vi "COMTRADE Read Private Inf (All Entries).vi"(8 "error in (no error)":errorcluster, 9 "section name":string, 10 "manufacturer name":string, 11 "task in":T1={"file refnums"=[], "Data Object"=refnum, "config info"={"station_name"="", "rec_dev_id"="", "rev_year"=1999.0, "TT"=0, "##A"=0, "##D"=0, "analog channel info"=[], "status channel info"=[], "lf"=50.0, "nrates"=0, "samp info"=[], "initial timestamp"=timestamp(0 s since 1904-01-01), "trigger timestamp"=timestamp(0 s since 1904-01-01), "ft"=enum."Binary", "timemult"=1.0}, "public inf content"={"Source"="", "Record Type"=enum."Unknown", "Phase ID"="", "Event Description"="", "Device ID"="", "Distance of Fault"=-1.0, "Distance Unit"=enum."Miles", "Max_Current"=inf, "Min_Current"=-inf, "Max_Voltage"=inf, "Min_Voltage"=-inf, "EventNoteCount"=0, "Event Information"=[]}, "private inf content"=[], "internal buffers"={"start index"=1, "config to public inf"=enum."disabled", "static config info"="", "static file_des record inf"="", "static file_des channel inf"="", "public inf"="", "private inf"=""}} {"public inf content"."Event Information"."min sample number" max=9999999999; "public inf content"."Event Information"."max sample number" max=9999999999; "config info"."nrates" max=999; "config info"."status channel info"."Dn" min=1 max=999999; "config info"."analog channel info"."An" min=1 max=999999; "config info"."trigger timestamp" format="%<%H:%M:%S%6u\n%d/%m/%Y>T"; "config info"."initial timestamp" format="%<%H:%M:%S%6u\n%d/%m/%Y>T"; "config info"."##D" max=999999; "config info"."##A" max=999999; "config info"."TT" min=1 max=999999; "config info"."rev_year" min=1999.0 max=1999.0}) -> (0 "error out":errorcluster, 1 "entry values":string[](array[string]), 2 "entry names":string[](array[string]), 3 "task out":T1={"file refnums"=[], "Data Object"=refnum, "config info"={"station_name"="", "rec_dev_id"="", "rev_year"=1999.0, "TT"=0, "##A"=0, "##D"=0, "analog channel info"=[], "status channel info"=[], "lf"=50.0, "nrates"=0, "samp info"=[], "initial timestamp"=timestamp(0 s since 1904-01-01), "trigger timestamp"=timestamp(0 s since 1904-01-01), "ft"=enum."Binary", "timemult"=1.0}, "public inf content"={"Source"="", "Record Type"=enum."Unknown", "Phase ID"="", "Event Description"="", "Device ID"="", "Distance of Fault"=-1.0, "Distance Unit"=enum."Miles", "Max_Current"=inf, "Min_Current"=-inf, "Max_Voltage"=inf, "Min_Voltage"=-inf, "EventNoteCount"=0, "Event Information"=[]}, "private inf content"=[], "internal buffers"={"start index"=1, "config to public inf"=enum."disabled", "static config info"="", "static file_des record inf"="", "static file_des channel inf"="", "public inf"="", "private inf"=""}} {"public inf content"."Event Information"."min sample number" max=9999999999; "public inf content"."Event Information"."max sample number" max=9999999999; "config info"."nrates" max=999; "config info"."status channel info"."Dn" min=1 max=999999; "config info"."analog channel info"."An" min=1 max=999999; "config info"."trigger timestamp" format="%<%H:%M:%S%6u\n%d/%m/%Y>T"; "config info"."initial timestamp" format="%<%H:%M:%S%6u\n%d/%m/%Y>T"; "config info"."##D" max=999999; "config info"."##A" max=999999; "config info"."TT" min=1 max=999999; "config info"."rev_year" min=1999.0 max=1999.0})   [LabVIEW 2013, in "NI_EP_COMTRADE.lvlib"]
doc: "Reads information from the private sections of the optionally specified .inf file. You must set <B>open mode</B> to Open (read only) in the COMTRADE Open VI to open the .inf file. Otherwise this VI returns an error."
uses:
  <vilib>/addons/Electrical Power/File IO/NI_EP_COMTRADE.lvlib
  <vilib>/addons/Electrical Power/File IO/COMTRADE/typedefs/ep_Task.ctl
  <vilib>/addons/Electrical Power/File IO/COMTRADE/typedefs/ep_Config Info.ctl
  <vilib>/addons/Electrical Power/File IO/COMTRADE/typedefs/ep_Analog Channel Info.ctl
  <vilib>/addons/Electrical Power/File IO/COMTRADE/typedefs/ep_Status Channel Info.ctl
  <vilib>/addons/Electrical Power/File IO/COMTRADE/typedefs/ep_File Format.ctl
  <vilib>/addons/Electrical Power/File IO/COMTRADE/typedefs/ep_Public Inf Content.ctl
  <vilib>/addons/Electrical Power/File IO/COMTRADE/typedefs/ep_Public Event Inf.ctl
  <vilib>/addons/Electrical Power/File IO/COMTRADE/typedefs/ep_Private Inf Content.ctl
  <vilib>/Platform/storage/Storage.llb/Get Property (Storage Refnums).vi
  <vilib>/Platform/storage/Storage.llb/Get Property (I32).vi
  <vilib>/Platform/storage/Storage.llb/Get Property (String).vi
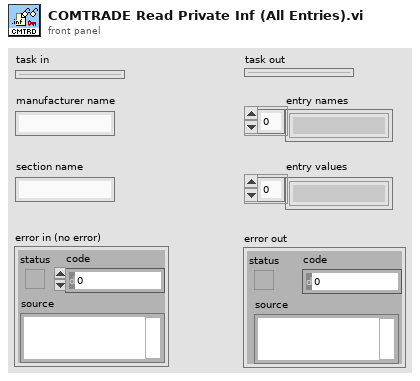
[diagram p1: front panel]
types:
  T1 = typedef "NI_EP_COMTRADE.lvlib/ep_Task.ctl" = cluster{"file refnums":refnum<file>[], "Data Object":refnum<k20>, "config info":T2, "public inf content":T6, "private inf content":T8, "internal buffers":cluster{"start index":u32, "config to public inf":enum16{"disabled", "enabled", "buffered"}, "static config info":string, "static file_des record inf":string, "static file_des channel inf":string, "public inf":string, "private inf":string}}
  T2 = typedef "NI_EP_COMTRADE.lvlib/ep_Config Info.ctl" = cluster{"station_name":string, "rec_dev_id":string, "rev_year":dbl, "TT":u32, "##A":u32, "##D":u32, "analog channel info":T3[], "status channel info":T4[], "lf":sgl, "nrates":u16, "samp info":cluster{"samp":sgl, "endsamp":u32}[], "initial timestamp":timestamp, "trigger timestamp":timestamp, "ft":T5, "timemult":sgl}
  T3 = typedef "NI_EP_COMTRADE.lvlib/ep_Analog Channel Info.ctl" = cluster{"An":u32, "ch_id":string, "ph":string, "ccbm":string, "uu":string, "a":sgl, "b":sgl, "skew":sgl, "min":i32, "max":i32, "primary":sgl, "secondary":sgl, "PS":enum16{"P", "S"}}
  T4 = typedef "NI_EP_COMTRADE.lvlib/ep_Status Channel Info.ctl" = cluster{"Dn":u32, "ch_id":string, "ph":string, "ccbm":string, "Y":bool}
  T5 = typedef "NI_EP_COMTRADE.lvlib/ep_File Format.ctl" = enum16{"ASCII", "Binary"}
  T6 = typedef "NI_EP_COMTRADE.lvlib/ep_Public Inf Content.ctl" = cluster{"Source":string, "Record Type":enum16{"Fault", "Unknown", "Misoperation", "Close", "Trip", "Reclose", "Power swing", "Simulation"}, "Phase ID":string, "Event Description":string, "Device ID":string, "Distance of Fault":dbl, "Distance Unit":enum16{"Miles", "Kilometers", "Percent of line", "Percent of setting", "Ohms"}, "Max_Current":dbl, "Min_Current":dbl, "Max_Voltage":dbl, "Min_Voltage":dbl, "EventNoteCount":u32, "Event Information":T7[]}
  T7 = typedef "NI_EP_COMTRADE.lvlib/ep_Public Event Inf.ctl" = cluster{"channel number":u32, "max value":dbl, "min value":dbl, "max sample number":u64, "min sample number":u64, "max sample text":string[], "min sample text":string[]}
  T8 = typedef "NI_EP_COMTRADE.lvlib/ep_Private Inf Content.ctl" = cluster{"Section Header":string, "Entry Names":string[], "Entry Values":string[]}[]
  T9 = typedef "usiProperty.ctl" = cluster{"object type":T10, "property name":string, "data type":T11}
  T10 = typedef "usiObjectType.ctl" = enum16{"File", "Channel Group", "Channel", "Unknown"}
  T11 = typedef "usiDataType.ctl" = enum16{"eNoTypeUsi", "eInt8Usi", "eInt16Usi", "eInt32Usi", "eInt64Usi", "eUInt8Usi", "eUInt16Usi", "eUInt32Usi", "eUInt64Usi", "eFloat32Usi", "eFloat64Usi", "- 0", "- 1", "- 2", "- 3", "- 4", "- 5", "- 6", "- 7", "- 8", "- 9", "eString8Usi", "eString16Usi", "eStringUsi", "eEnumUsi", "- 10", "- 11", "- 12", "- 13", "- 14", "eTimeUsi", "- 15", "- 16", "- 17", "- 18", "- 19", "- 20", "- 21", "- 22", "- 23", "eInstanceUsi", "eStoreUsi"}
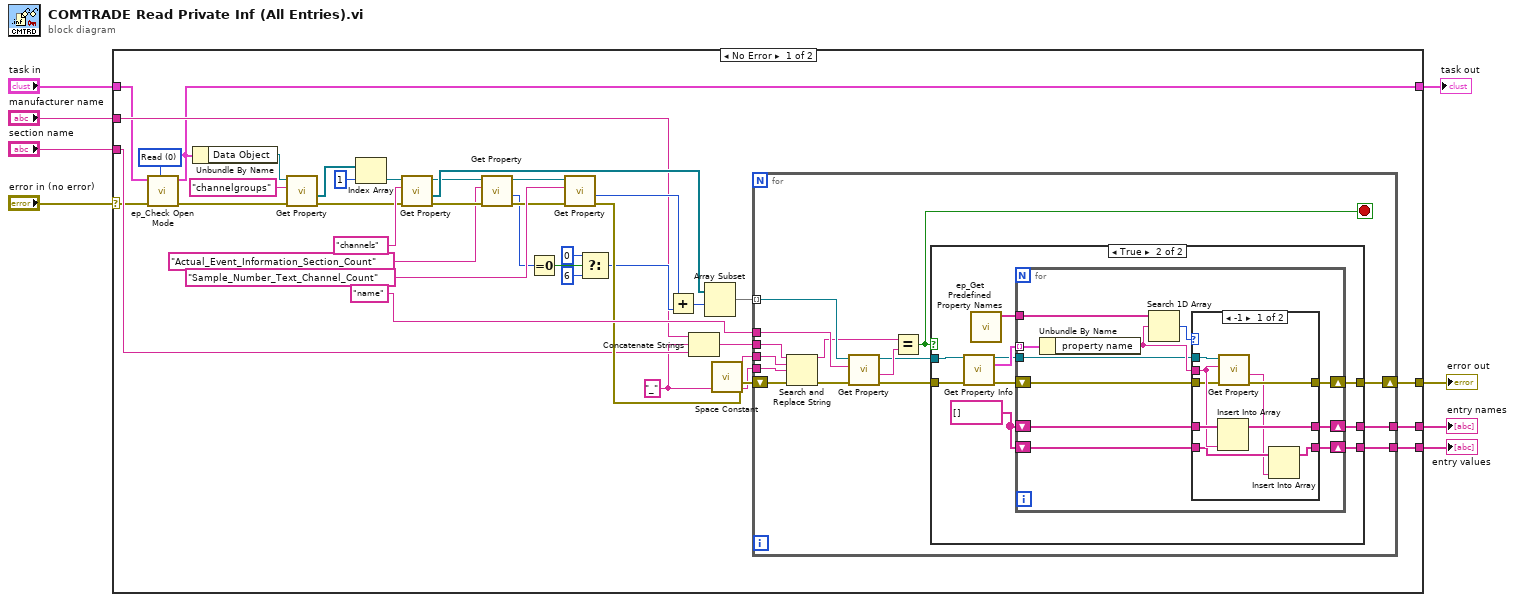
[diagram p0: block diagram]
diagram:
  n1 = case shown="No Error" "error in (no error)" {
    selector: "error in (no error)" -> [w12 w95]
    tunnel: "task in" -> [w10 w96]
    tunnel: [w9 w96] -> w3
    tunnel: [w29 w95] -> w7
    tunnel: "manufacturer name" -> [w18 _]
    tunnel: "section name" -> [w31 _]
    tunnel: [w15 _] -> w1
    tunnel: [w14 _] -> w2
    frame No Error {
      w13 = u16 0 items=["Read", "Write"] ("file type")
      w16 = "_" ("string")
      n2 = call <vilib>:"ep_Check Open Mode.vi"("expected mode"=w13, "error in (no error)"=w12, "task in"=w10) -> ("error out"=w11:errorcluster, "task out"=w9:T1)  [unwired: 7 in]
      n3 = Unbundle By Name(w9) -> ("Data Object"=w45:refnum<k20>)
      n4 = call-poly <vilib>:"Get Property.vi"("error in (no error)"=w11, "Property name"="channelgroups", "storage refnum"=w45) -> ("error out"=w35:errorcluster, "Value"=w44:refnum<k20>[])  [unwired: 6 in, 1 out]
      n5 = Index Array(array=w44, index=1) -> (element=w40:refnum<k20>)
      n6 = call-poly <vilib>:"Get Property.vi"("error in (no error)"=w35, "Property name"="channels", "storage refnum"=w40) -> ("error out"=w28:errorcluster, "Value"=w39:refnum<k20>[], "storage refnum out"=w20:refnum<k20>)  [unwired: 6 in]
      n7 = call-poly <vilib>:"Get Property.vi"("error in (no error)"=w28, "Property name"="Actual_Event_Information_Section_Count", "storage refnum"=w20) -> ("error out"=w27:errorcluster, "Value"=w24:i32, "storage refnum out"=w19:refnum<k20>)  [unwired: 6 in]
      n8 = Equal To 0?(x=w24) -> (x = 0?=w25:bool)
      n9 = call-poly <vilib>:"Get Property.vi"("error in (no error)"=w27, "Property name"="Sample_Number_Text_Channel_Count", "storage refnum"=w19) -> ("error out"=w32:errorcluster, "Value"=w37:i32)  [unwired: 6 in, 1 out]
      n10 = Select(t=0 ("index"), s=w25, f=6 ("index")) -> (s? t:f=w23:i32)
      n11 = Add(x=w37, y=w23) -> (x+y=w38:i32)
      n12 = Concatenate Strings(w18, w16, w31) -> (w30:string)
      n13 = Array Subset(array=w39, index=w38) -> (w34:refnum<k20>[])  [unwired: 1 in]
      n14 = call <vilib>:"Space Constant.vi"() -> ("String"=w17:string)
      n15 = for {
        tunnel: w34 -> [w60] mode=indexing
        tunnel: "name" ("Property name") -> [w59]
        shift-right: [w47] -> w29
        shift-left: w32 -> [w51]
        tunnel: w30 -> [w54]
        tunnel: w17 -> [w53]
        tunnel: w16 -> [w52]
        tunnel: [w48] -> w15
        tunnel: [w46] -> w14
        stop <- w55 stop-if-true
        n16 = Search and Replace String(input string=w54, search string=w53, replace string=w52, error in=w51) -> (result string=w49:string, error out=w50:errorcluster)  [unwired: 4 in, 2 out]
        n17 = call-poly <vilib>:"Get Property.vi"("error in (no error)"=w50, "Property name"=w59, "storage refnum"=w60) -> ("error out"=w56:errorcluster, "Value"=w58:string, "storage refnum out"=w57:refnum<k20>)  [unwired: 6 in]
        n18 = Equal?(x=w49, y=w58) -> (x = y?=w55:bool)
        n19 = case shown="True" w55 {
          tunnel: w57 -> [_ w68]
          tunnel: w56 -> [w61 w71]
          tunnel: [w61 w64] -> w47
          tunnel: [_ w63] -> w48
          tunnel: [_ w67] -> w46
          frame False {
          }
          frame True {
            w62 = string[] [] ("pre-defined property names")
            n20 = call <vilib>:"Get Property Info.vi"("storage refnum"=w68, "error in (no error)"=w71) -> ("storage refnum out"=w66:refnum<k20>, "properties"=w70:T9[], "error out"=w65:errorcluster)  [unwired: 11 in]
            n21 = call <vilib>:"ep_Get Predefined Property Names.vi"() -> ("pre-defined property names"=w69:string[])  [unwired: 11 in]
            n22 = for {
              tunnel: w70 -> [w82] mode=indexing
              tunnel: w69 -> [w81]
              shift-right: [w77] -> w67
              shift-left: w62 -> [w79]
              tunnel: w66 -> [w74]
              shift-right: [w72] -> w64
              shift-left: w65 -> [w73]
              shift-right: [w75] -> w63
              shift-left: w62 -> [w76]
              n23 = Unbundle By Name(w82) -> ("property name"=w78:string)
              n24 = Search 1D Array(1D array=w81, element=w78) -> (index of element=w80:i32)  [unwired: 1 in]
              n25 = case shown="-1" w80 {
                tunnel: w79 -> [w91 w94]
                tunnel: [w90 w94] -> w77
                tunnel: w78 -> [w88 _]
                tunnel: w76 -> [w85 w93]
                tunnel: [w83 w93] -> w75
                tunnel: w74 -> [w89 _]
                tunnel: w73 -> [w87 w92]
                tunnel: [w86 w92] -> w72
                frame -1 {
                  n26 = Insert Into Array(array=w91, new element=w88) -> (w90:string[])  [unwired: 1 in]
                  n27 = call-poly <vilib>:"Get Property.vi"("error in (no error)"=w87, "Property name"=w88, "storage refnum"=w89) -> ("error out"=w86:errorcluster, "Value"=w84:string)  [unwired: 6 in, 1 out]
                  n28 = Insert Into Array(array=w85, new element=w84) -> (w83:string[])  [unwired: 1 in]
                }
                frame Default {
                }
              }
            }
          }
        }
      }
    }
    frame Error {
    }
  }
  "error out" <- w7
  "entry values" <- w1
  "task out" <- w3
  "entry names" <- w2
